vi "Client Spawn.vi"(8 "Log Instance":refnum<class "LoggerReference.lvclass">, 9 "Return Queue":refnum<queue>, 10 "User Event":refnum<user-event>, 11 "Client ID":string) -> ()   [LabVIEW 2019, in "Network Logger Examples.lvlib"]
uses:
  <vilib>/gpm_packages/@cs/event-logger/Examples/Examples/Network Logger Examples.lvlib
  <vilib>/gpm_packages/@cs/event-logger/Source/Composed Log/LoggerReference/LoggerReference.lvclass
  <vilib>/gpm_packages/@cs/event-logger/Examples/Examples/BasicNetworkProtocol/BasicNetworkProtocol.lvclass
  C:/Program Files/National Instruments/LabVIEW 2019/vi.lib/gpm_packages/@cs/Network-Sink/Source/Network Interface/IMessagingProtocol/IMessagingProtocol.lvclass
  <vilib>/gpm_packages/@cs/Network-Sink/Source/Network Interface/Network Interface/Network Interface.lvclass/Network Interface.ctl
  <vilib>/gpm_packages/@cs/Network-Sink/Source/Network Interface/Message Queue/Message Queue.lvclass/Message Queue.ctl
  <vilib>/gpm_packages/@cs/Network-Sink/Source/Network Interface/Network Interface/Write.vi/dc351019-4f29-47b2-a483-8ae26d0321a6.vi
  <vilib>/gpm_packages/@cs/Network-Sink/Source/Network Interface/Message Queue/Protected Enqueue.vi
  <vilib>/gpm_packages/@cs/Network-Sink/Source/TCP Interface/TCP Client/TCP Client.lvclass
  C:/Program Files/National Instruments/LabVIEW 2019/vi.lib/gpm_packages/@cs/Network-Sink/Source/Network Interface/IConnectionFactory/IConnectionFactory.lvclass
  <vilib>/gpm_packages/@cs/Network-Sink/Source/Network Interface/Network Interface/Network Interface.lvclass
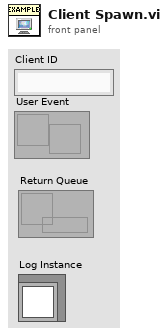
[diagram p1: front panel]
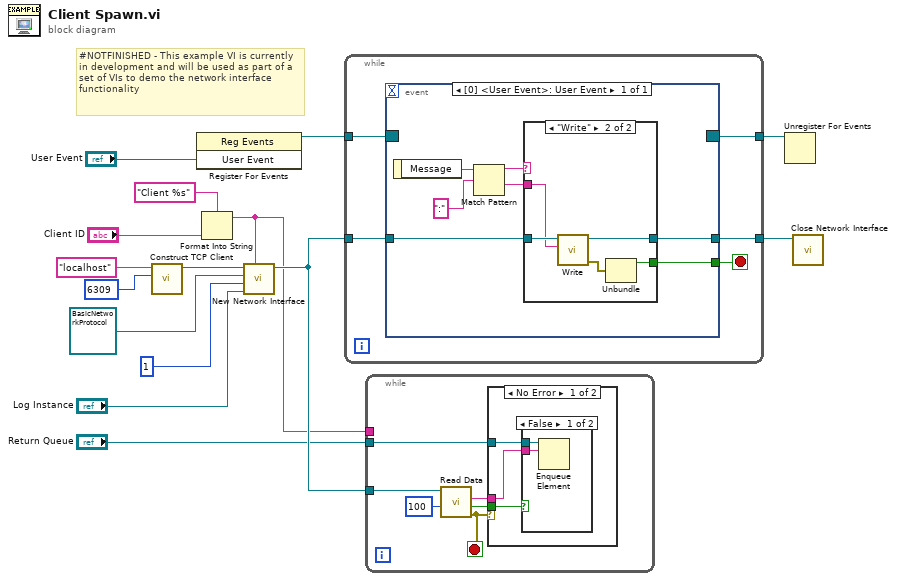
[diagram p0: block diagram]
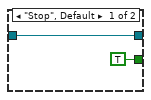
[diagram p4: hidden frame]
diagram:
  # "#NOTFINISHED - This example VI is currently in development and will be used as part of a set of VIs to demo the network interface functionality"
  n1 = call <vilib>:"Construct TCP Client.vi"("Remote Port or Service Name"=u16 6309 ("Local Port (0)"), "Address"="localhost") -> ("TCP Client out"=w15:refnum<class "TCP Client.lvclass">)  [unwired: 9 in]
  n2 = register-events("User Event") -> (reference out=w6:refnum<event-registration>)  [unwired: 2 in, 1 out]
  n3 = Format Into String(format string="Client %s", "Client ID") -> (resulting string=w1:string)  [unwired: 2 in, 1 out]
  n4 = call <vilib>:"New Network Interface.vi"("Log Alias"=w1, "Log Instance"="Log Instance", "Max Number of Connections to Create (1)"=1 ("Max Number of Connections"), "MessageProtocol"=refnum<class "BasicNetworkProtocol.lvclass"> refnum ("BasicNetworkProtocl.lvclass"), "Connection Factory Type"=w15) -> ("Network Interface Reference"=w8:refnum<data-value>)  [unwired: 5 in, 1 out]
  n5 = while {
    tunnel: w8 -> [w20]
    tunnel: w6 -> [w19]
    tunnel: [w18] -> w3
    tunnel: [w16] -> w4
    stop <- w17 stop-if-true
    n6 = event shown="[0] <User Event>: User Event" {
      selector: w19 -> [_]
      dyn-events: [_] -> w16
      timeout: _ -> [_]
      tunnel: w20 -> [w27]
      tunnel: [w22] -> w18
      tunnel: [w21] -> w17
      event User Event {
        n7 = event-data() -> ("Message"=w26:string)  [unwired: 1 in]
        n8 = Match Pattern(string=w26, regular expression=":") -> (before substring=w24:string, after substring=w23:string)  [unwired: 1 in, 2 out]
        n9 = case shown="\"Write\"" w24 {
          tunnel: w27 -> [w29 w34]
          tunnel: w23 -> [_ w33]
          tunnel: [TRUE ("status") w30] -> w21
          tunnel: [w29 w32] -> w22
          frame "Stop", Default {
          }
          frame "Write" {
            n10 = call <vilib>:"Write.vi"("Data To Write"=w33, "Network Interface"=w34) -> ("error out"=w31:errorcluster, "Network Interface Out"=w32:refnum<data-value>)  [unwired: 8 in]
            n11 = Unbundle(w31) -> ("status"=w30:bool)  [unwired: 2 out]
          }
        }
      }
    }
  }
  n12 = while {
    tunnel: w8 -> [w40]
    tunnel: "Return Queue" -> [w38]
    tunnel: w1 -> [_]
    stop <- w35 stop-if-true
    n13 = call <vilib>:"Read Data.vi"("Timeout in ms (-1)"=100, "Network Interface"=w40) -> ("error out"=w35:errorcluster, "Timed Out?"=w36:bool, "Read Data"=w37:string)  [unwired: 6 in, 1 out]
    n14 = case shown="No Error" w35 {
      tunnel: w38 -> [w43 _]
      tunnel: w37 -> [w42 _]
      tunnel: w36 -> [w41 _]
      frame No Error {
        n15 = case shown="False" w41 {
          tunnel: w43 -> [w45 _]
          tunnel: w42 -> [w44 _]
          frame False {
            n16 = Enqueue Element(queue=w45, element=w44) -> ()  [unwired: 2 in, 3 out]
          }
          frame True {
          }
        }
      }
      frame Error {
      }
    }
  }
  n17 = Unregister For Events(event registration refnum=w4) -> ()  [unwired: 1 in, 1 out]
  n18 = call <vilib>:"Close Network Interface.vi"("Network Interface"=w3) -> ()  [unwired: 10 in, 1 out]
